vi "FT_Set_Data_Characteristics.vi"(1 "Parity":u8(ring) items=["FT_PARITY_NONE", "FT_PARITY_ODD", "FT_PARITY_EVEN", "FT_PARITY_MARK", "FT_PARITY_SPACE"], 2 "Stop Bits":u8(ring) items=["FT_STOP_BITS_1"=0, "FT_STOP_BITS_2"=2], 3 "Word Length":u8(ring)=8 items=["FT_BITS_7"=7, "FT_BITS_8"=8], 4 "Handle":u32) -> (0 "FT_Status":u32)   [LabVIEW 2013]
uses:
  FTD2XX.dll
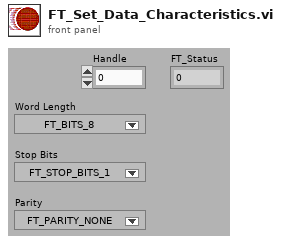
[diagram p1: front panel]
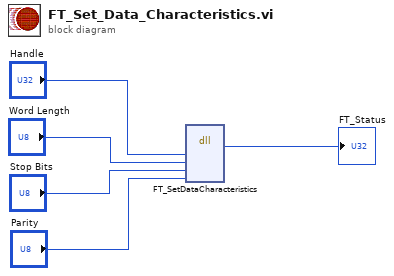
[diagram p0: block diagram]
diagram:
  n1 = dll-call lib="FTD2XX.dll" fn="FT_SetDataCharacteristics" label="FT_SetDataCharactceristics"("Handle"="Handle", "WordLength"="Word Length", "StopBits"="Stop Bits", "Parity"="Parity") -> ("FT_Status"=→"FT_Status":u32)  [unwired: 7 in, 2 out]
